vi "OE2052_Query PLL&Overload.vi"(0 "VISA resource name":refnum<visa-resource-name>, 1 "Timeout":u32=1000, 5 "Connection ID in":refnum<k5>, 7 "channel":u16(ring)=1 items=["A"=1, "B"=2], 9 "Remote Mode":u16(ring) items=["USB"=0, "RS232"=1, "Ethernet"=3], 11 "Error in (no error)":errorcluster caption="error out（no error）") -> (4 "VISA resource  out":refnum<visa-resource-name>, 6 "Connection ID out":refnum<k5>, 8 "OE2052_Query \nPLL&Overload":cluster{"PLL Lock":bool, "Overload":bool}, 10 "Output String":string, 15 "Error out":errorcluster caption="error out")   [LabVIEW 2011]
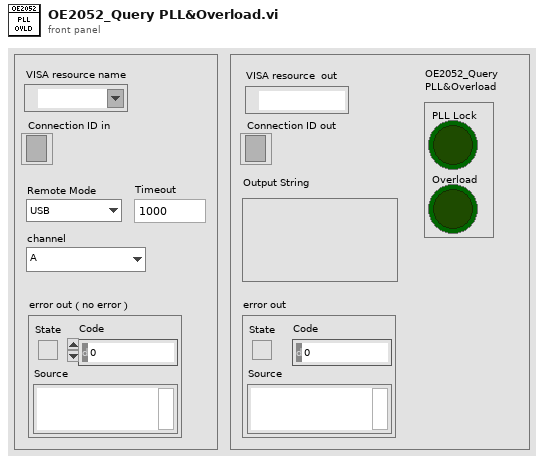
[diagram p1: front panel]
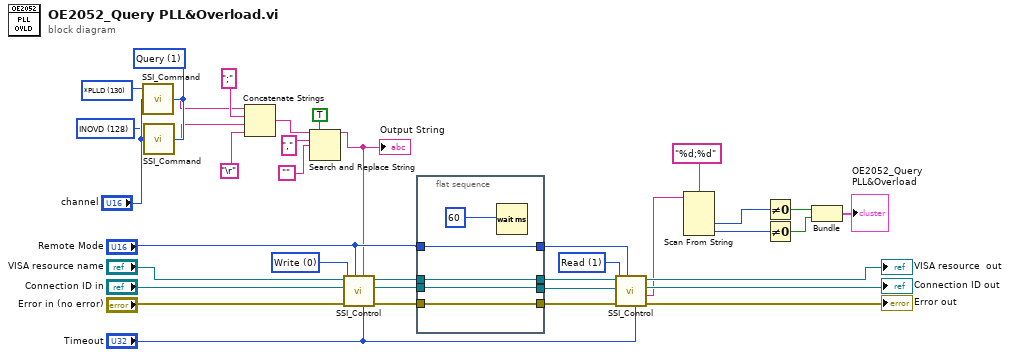
[diagram p0: block diagram]
diagram:
  w15 = u16 130 items=["ISRC", "IGND", "ICPL", "ILIN", "PHAS", "FMOD", "RSLP", "FREQ", "SWPT", "SLLM", "SULM", "SSLL", "SSLG", "STLM", "SWRM", "IRNG", "SENS", "RMOD", "OFLT", "OFSL", "SYNC", "DMOD", "HARM", "DARB", "SWVT", "SLVL", "SVLL", "SVUL", "SVSL", "SVSG", "SVTM", "SVRM", "RALL", "SNAP", "OUTP", "OAUX", "COUT", "CAUX", "COFP", "CEXP", "FPOP", "OEXP", "*IDN", "*RST", "OVLD", "INOV", "GNOV", "*PLL", "SSET", "RSET", "AGAN", "APHS", "ARSV", "ASCL", "EQCD", "EQCS", "SPED", "SRAT", "SLEN", "SSLE", "STRG", "SPRM", "STRD", "PAUS", "REST", "SPTS", "TRCA", "TEMP", "RSTU", "INHZ", "DEQU", "SADD", "ARNG", "CSPE", "ISRCD", "IGNDD", "ICPLD", "ILIND", "PHASD", "FMODD", "RSLPD", "FREQD", "SWPTD", "SLLMD", "SULMD", "SSLLD", "SSLGD", "STLMD", "SWRMD", "SENSD", "RMODD", "OFLTD", "OFSLD", "SYNCD", "HARMD", "EQCDD", "EQCSD", "SNAPD", "OUTPD", "SWVTD", "SLVLD", "SVLLD", "SVULD", "SVSLD", "SVSGD", "SVTMD", "SVRMD", "SVDCD", "ARSVD", "AGAND", "APHSD", "ASCLD", "FPOPD", "CAUXD", "OEXPD", "SPEDD", "SRATD", "SLEND", "SSLED", "STRGD", "SPRMD", "STRDD", "PAUSD", "RESTD", "SPTSD", "TRCAD", "*IDND", "*RSTD", "INOVD", "GNOVD", "*PLLD", "SSETD", "RSETD", "RALLD", "NIPA", "NSMA", "NGWA", "NMAC", "NMOD", "TRIG", "TRCB", "INHZD", "ISAMD", "IRAGD", "RRAGD", "SOFFD", "DMODD", "COUTD", "COFPD", "CEXPD", "ARNGD", "OAUXD", "TRIM", "SUITD", "SNHZD", "AOFSD"] ("Command Type")
  w16 = u16 128 items=["ISRC", "IGND", "ICPL", "ILIN", "PHAS", "FMOD", "RSLP", "FREQ", "SWPT", "SLLM", "SULM", "SSLL", "SSLG", "STLM", "SWRM", "IRNG", "SENS", "RMOD", "OFLT", "OFSL", "SYNC", "DMOD", "HARM", "DARB", "SWVT", "SLVL", "SVLL", "SVUL", "SVSL", "SVSG", "SVTM", "SVRM", "RALL", "SNAP", "OUTP", "OAUX", "COUT", "CAUX", "COFP", "CEXP", "FPOP", "OEXP", "*IDN", "*RST", "OVLD", "INOV", "GNOV", "*PLL", "SSET", "RSET", "AGAN", "APHS", "ARSV", "ASCL", "EQCD", "EQCS", "SPED", "SRAT", "SLEN", "SSLE", "STRG", "SPRM", "STRD", "PAUS", "REST", "SPTS", "TRCA", "TEMP", "RSTU", "INHZ", "DEQU", "SADD", "ARNG", "CSPE", "ISRCD", "IGNDD", "ICPLD", "ILIND", "PHASD", "FMODD", "RSLPD", "FREQD", "SWPTD", "SLLMD", "SULMD", "SSLLD", "SSLGD", "STLMD", "SWRMD", "SENSD", "RMODD", "OFLTD", "OFSLD", "SYNCD", "HARMD", "EQCDD", "EQCSD", "SNAPD", "OUTPD", "SWVTD", "SLVLD", "SVLLD", "SVULD", "SVSLD", "SVSGD", "SVTMD", "SVRMD", "SVDCD", "ARSVD", "AGAND", "APHSD", "ASCLD", "FPOPD", "CAUXD", "OEXPD", "SPEDD", "SRATD", "SLEND", "SSLED", "STRGD", "SPRMD", "STRDD", "PAUSD", "RESTD", "SPTSD", "TRCAD", "*IDND", "*RSTD", "INOVD", "GNOVD", "*PLLD", "SSETD", "RSETD", "RALLD", "NIPA", "NSMA", "NGWA", "NMAC", "NMOD", "TRIG", "TRCB", "INHZD", "ISAMD", "IRAGD", "RRAGD", "SOFFD", "DMODD", "COUTD", "COFPD", "CEXPD", "ARNGD", "OAUXD", "TRIM", "SUITD", "SNHZD", "AOFSD"] ("Command Type")
  w26 = u16 1 items=["Write", "Read"] ("Control")
  w25 = u16 1 items=["Set", "Query"] ("Opera")
  w36 = u16 0 items=["Write", "Read"] ("Control")
  n1 = call "SSI_Command.vi"("Opera"=w25, "channel"="channel", "Command Type"=w15) -> ("Output string"=w3:string)  [unwired: 1 in]
  n2 = call "SSI_Command.vi"("Opera"=w25, "channel"="channel", "Command Type"=w16) -> ("Output string"=w2:string)  [unwired: 1 in]
  n3 = Concatenate Strings(w3, ";", w2, "\r") -> (w7:string)
  n4 = Search and Replace String(replace all?=TRUE ("替换全部？(F)"), input string=w7, search string="," ("搜索字符串"), replace string="") -> (result string=w1:string)  [unwired: 4 in, 3 out]
  "Output String" <- w1
  n5 = call "SSI_Control.vi"("Tineout"="Timeout", "Write Buffer"=w1, "Remote Mode"="Remote Mode", "Error in (no error)"="Error in (no error)", "Control"=w36, "Connection ID in"="Connection ID in", "VISA resource name"="VISA resource name") -> ("Error out"=w34:errorcluster, "Connection ID out"=w20:refnum<k5>, "VISA resource  out"=w33:refnum<visa-resource-name>)  [unwired: 1 in, 1 out]
  n6 = flat-sequence {
    tunnel: [w42] -> w32
    tunnel: w34 -> [w42]
    tunnel: [w41] -> w31
    tunnel: w33 -> [w41]
    tunnel: "Remote Mode" -> [w40]
    tunnel: [w40] -> w30
    tunnel: w20 -> [w39]
    tunnel: [w39] -> w19
    frame #0 {
      n7 = Wait (ms)(milliseconds to wait=u32 60 ("等待时间（毫秒）")) -> ()  [unwired: 1 out]
    }
  }
  n8 = call "SSI_Control.vi"("Tineout"="Timeout", "Remote Mode"=w30, "Error in (no error)"=w32, "Control"=w26, "Connection ID in"=w19, "VISA resource name"=w31) -> ("Error out"=→"Error out":errorcluster, "Read Buffer"=w13:string, "Connection ID out"=→"Connection ID out":refnum<k5>, "VISA resource  out"=→"VISA resource  out":refnum<visa-resource-name>)  [unwired: 2 in]
  n9 = Scan From String(format string="%d;%d" ("格式字符串"), input string=w13) -> (output 1=w12:i32, output 2=w11:i32)  [unwired: 4 in, 3 out]
  n10 = Not Equal To 0?(x=w12) -> (x != 0?=w27:bool)
  n11 = Not Equal To 0?(x=w11) -> (x != 0?=w24:bool)
  n12 = Bundle(w27, w24) -> (→"OE2052_Query \nPLL&Overload":cluster{bool, bool})  [unwired: 1 in]
